vi "EXDIR-YAML_Parse_Exdir.vi"() -> ()   [LabVIEW 2016]
uses:
  <vilib>/NI/Tree/Tree Manager/Tree.lvclass
panel:
  out "substring before match":string
  in  "stop":bool
  in  "OK":bool
  in  "Tree":string(tree)
  out "text":string
  in  "file (use dialog)":path
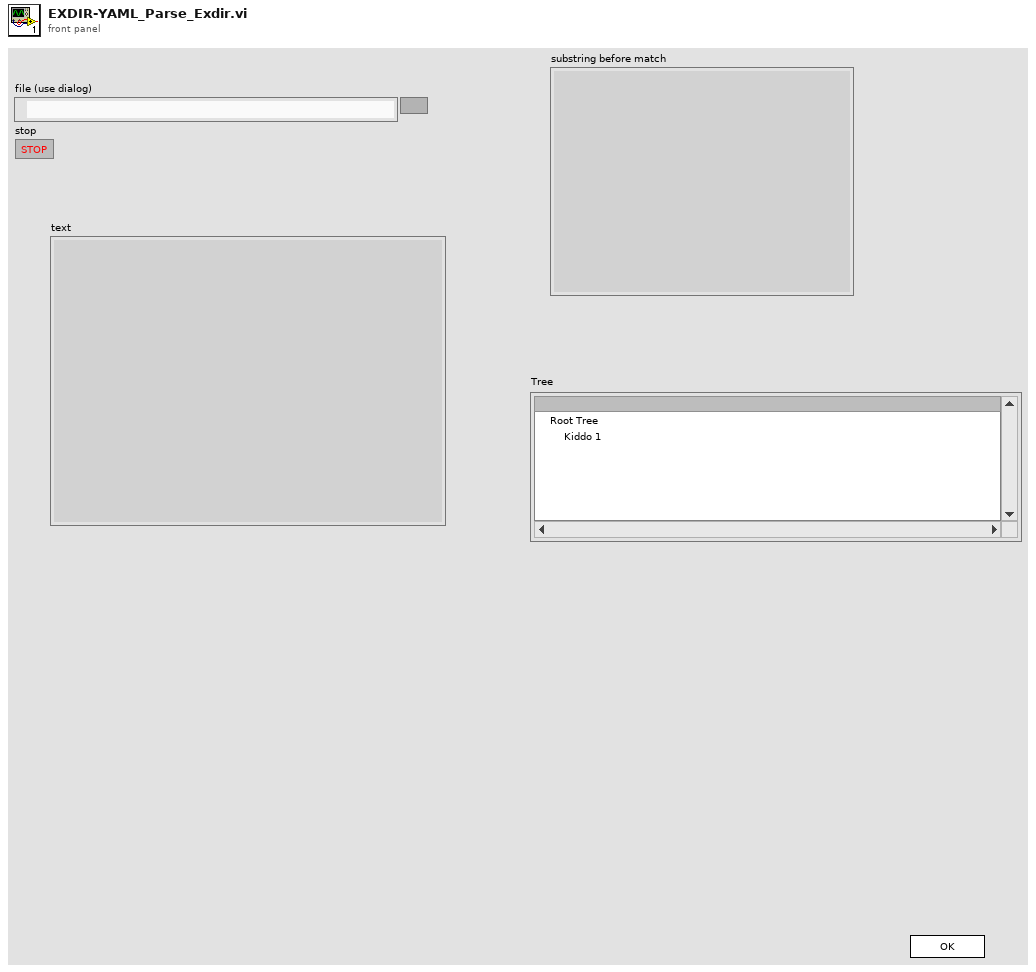
[diagram p1: front panel]
types:
  T1 = enum32{"invalid app kind", "Development System", "Run Time System", "Student Edition", "Embedded LabVIEW", "Evaluation", "Custom"}
  T2 = enum32{"Invalid", "Standard", "Closed", "Hidden", "Minimized", "Maximized"}
  T3 = cluster{"Core":cluster{"Current VI Reference":refnum<vi>, "Close Panel on Exit?":bool}, "Tree Manager":refnum<data-value>, "Unique ID":string, "Value":path, "Full YAML String":string, "queue out":refnum<queue>}
  T4 = cluster{"Current VI Reference":refnum<vi>, "Close Panel on Exit?":bool}
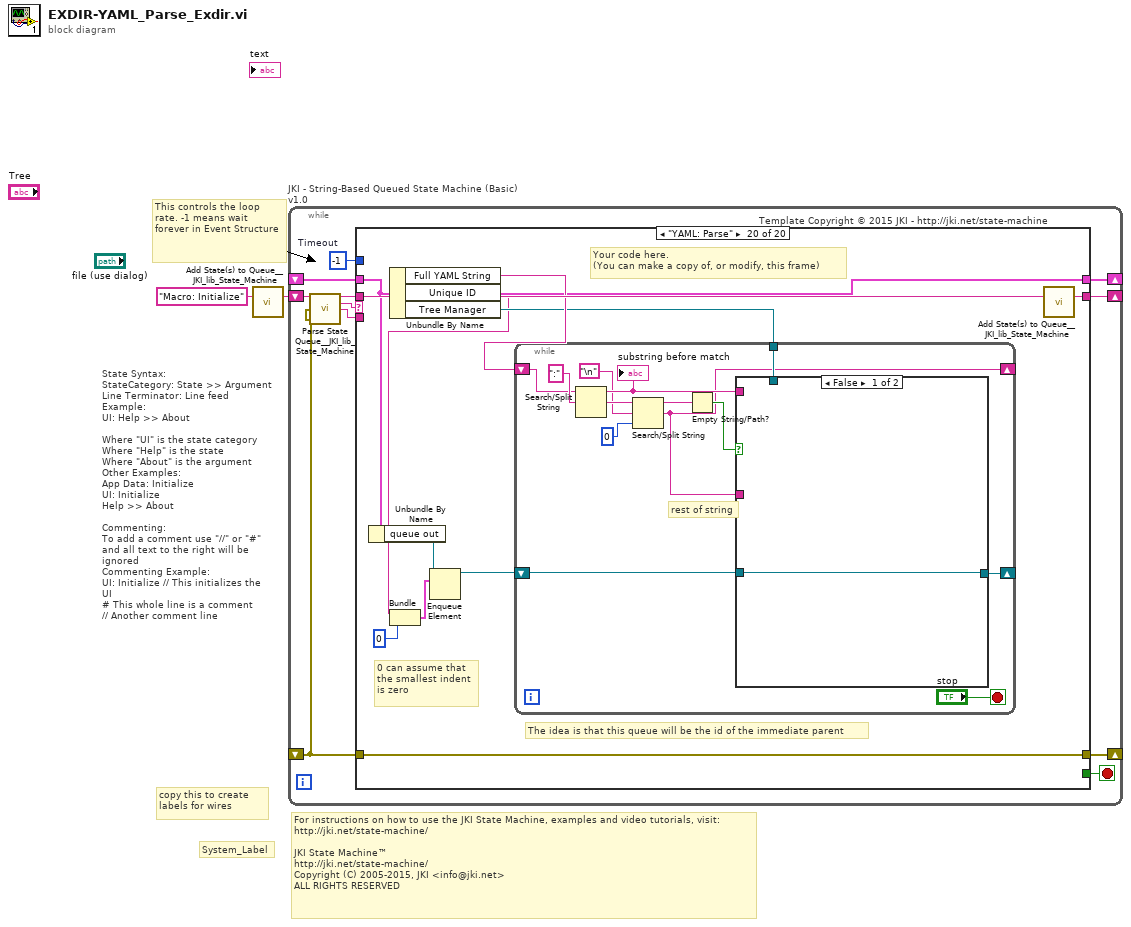
[diagram p0: block diagram]
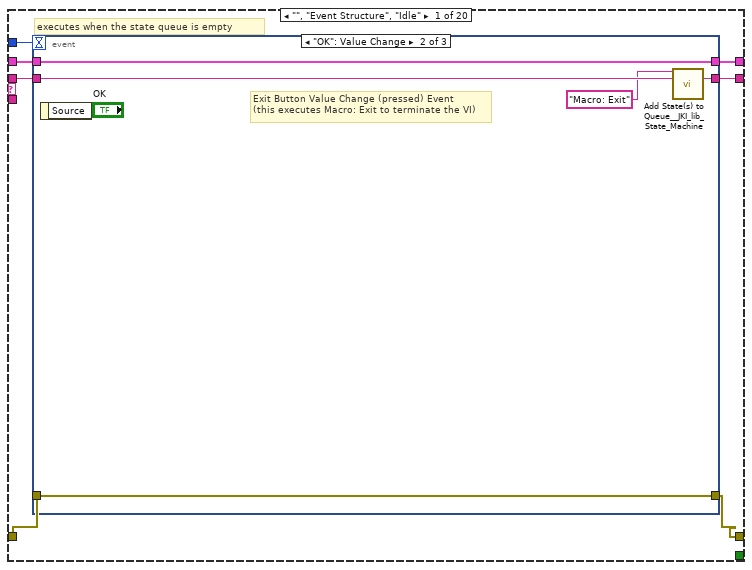
[diagram p2: hidden frame]
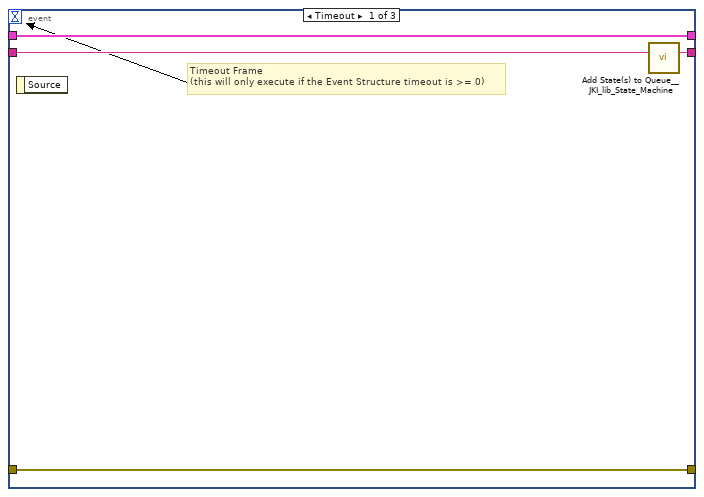
[diagram p3: hidden frame]
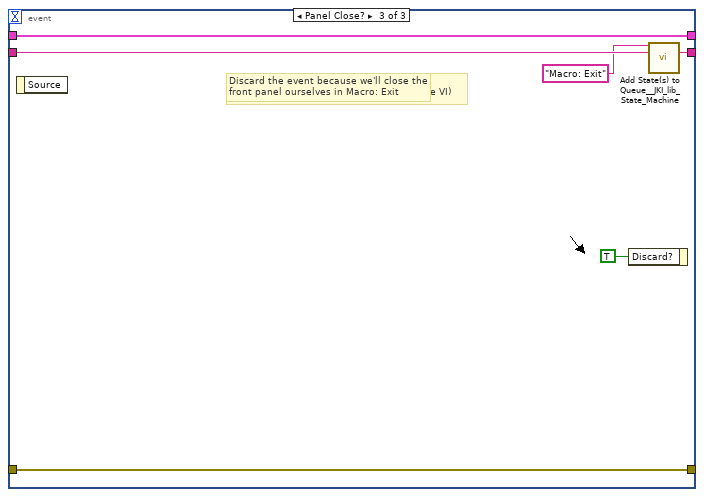
[diagram p4: hidden frame]
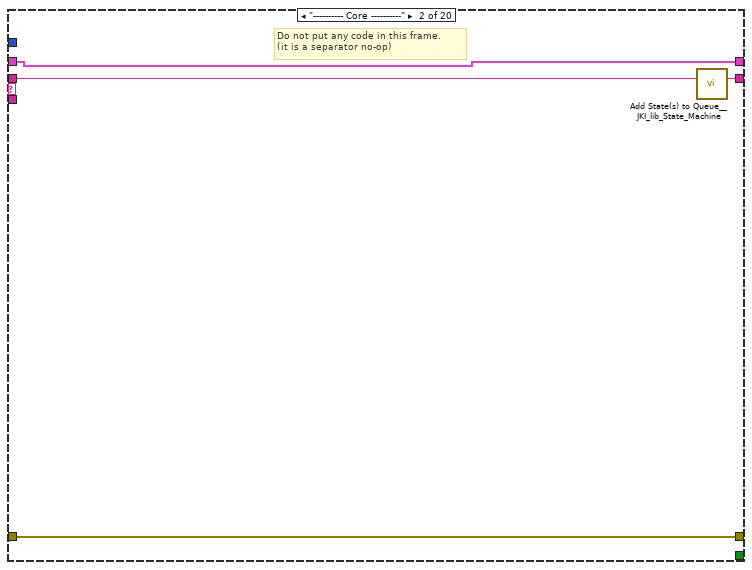
[diagram p5: hidden frame]
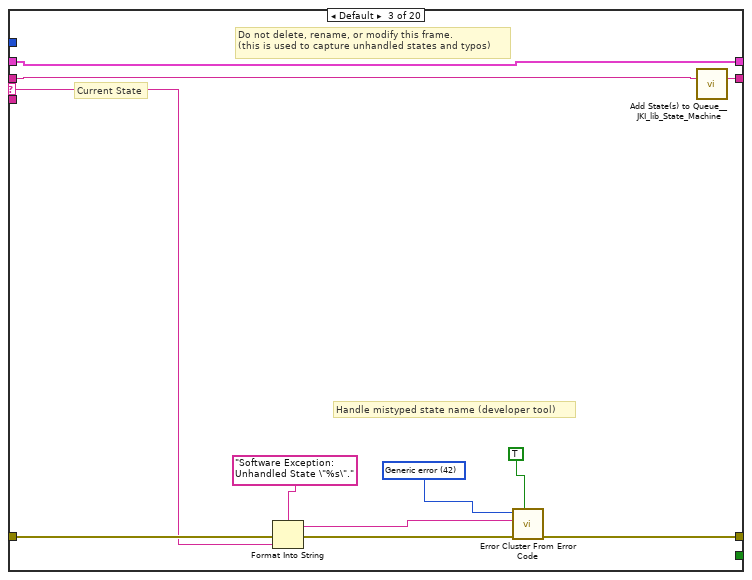
[diagram p6: hidden frame]
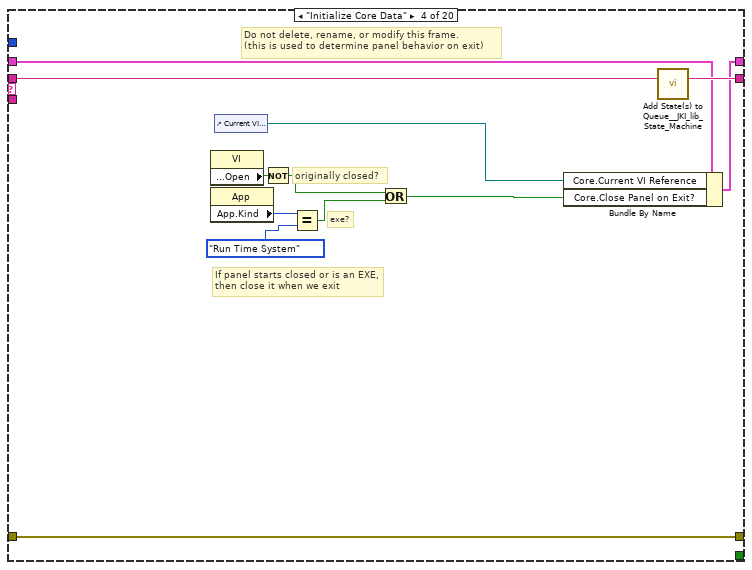
[diagram p7: hidden frame]
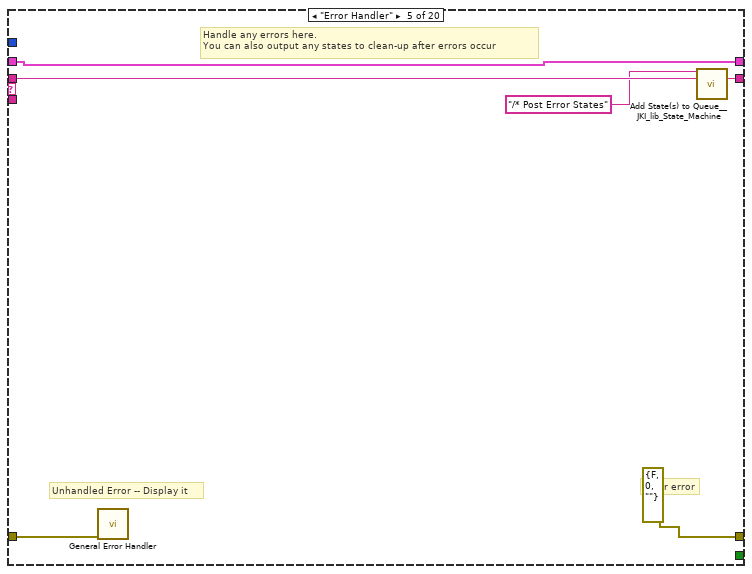
[diagram p8: hidden frame]
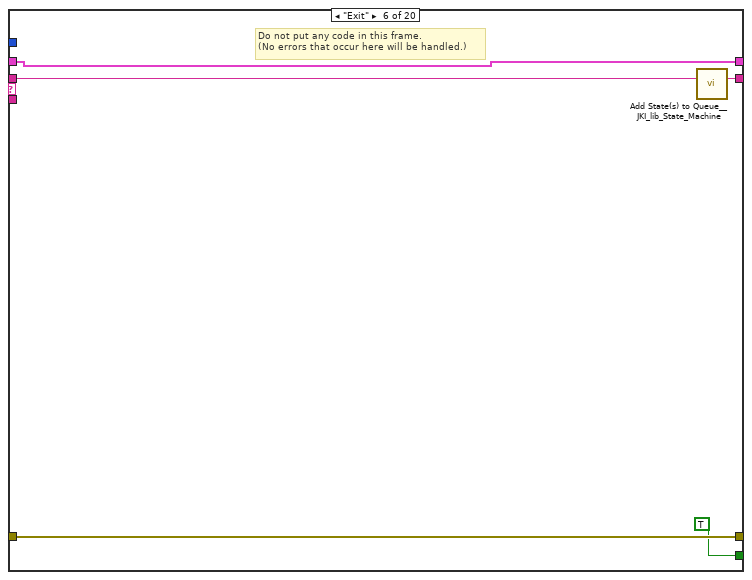
[diagram p9: hidden frame]
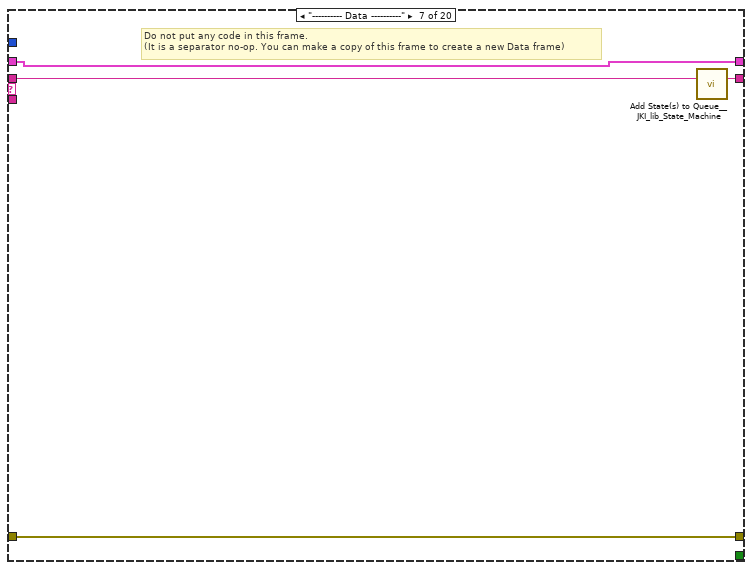
[diagram p10: hidden frame]
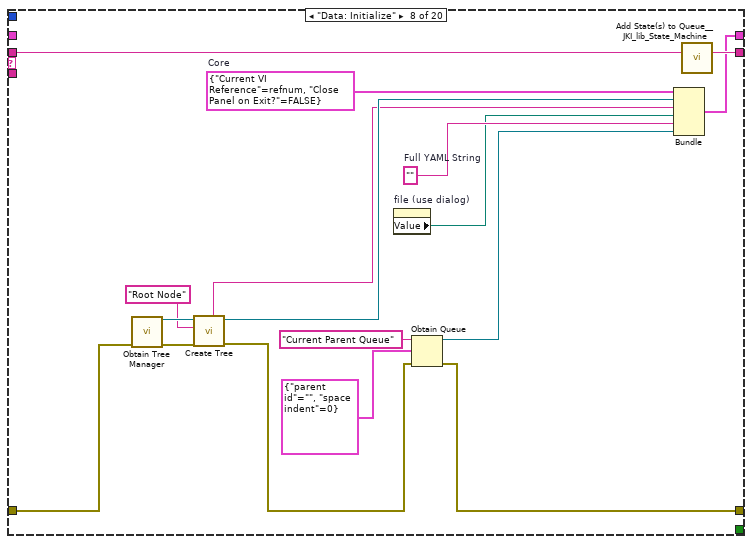
[diagram p11: hidden frame]
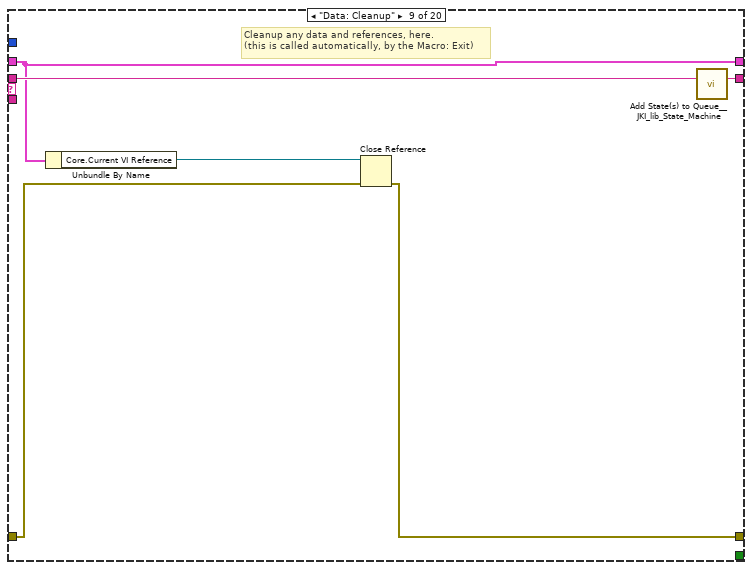
[diagram p12: hidden frame]
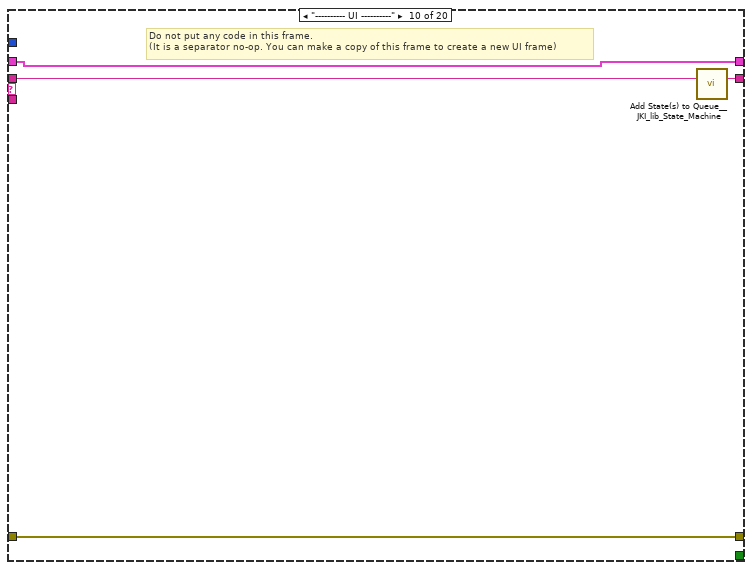
[diagram p13: hidden frame]
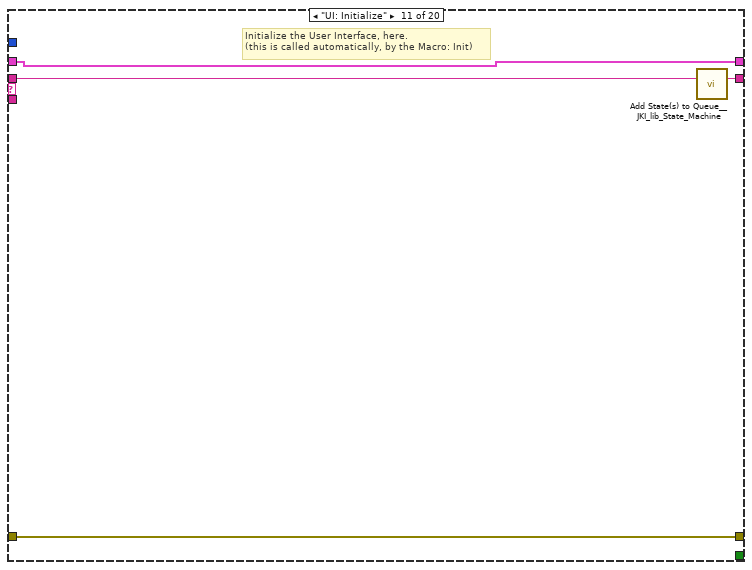
[diagram p14: hidden frame]
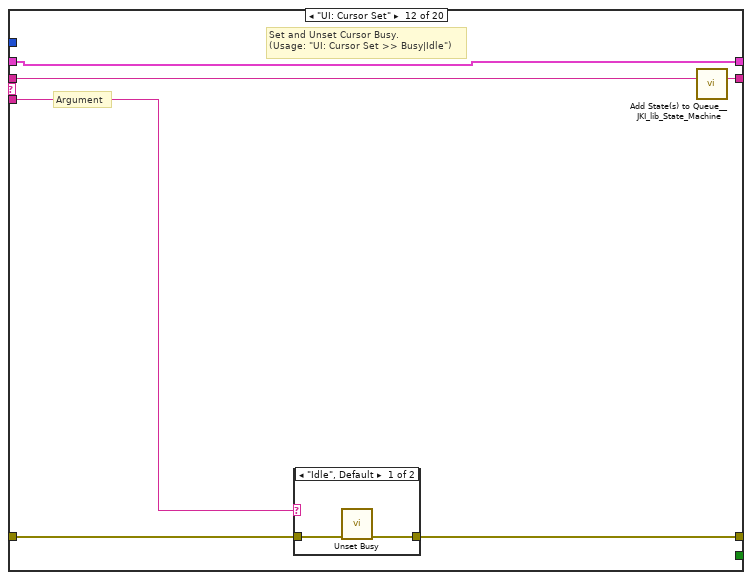
[diagram p15: hidden frame]
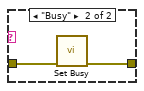
[diagram p16: hidden frame]
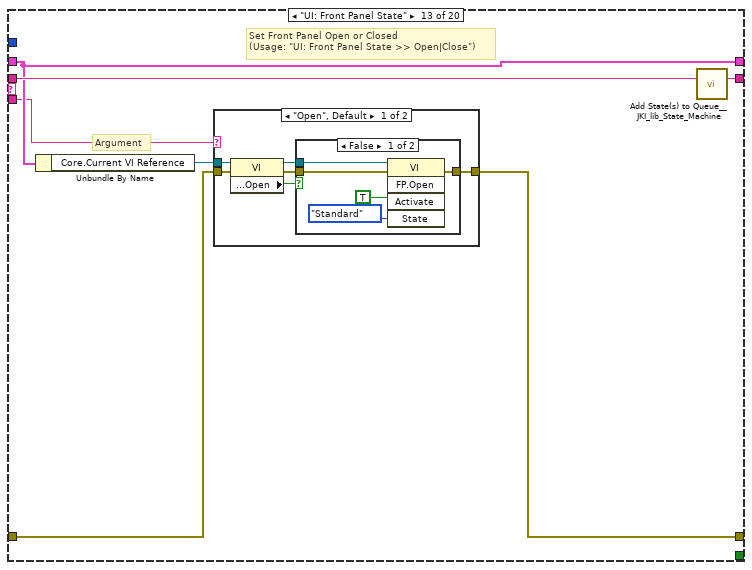
[diagram p17: hidden frame]
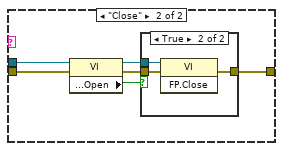
[diagram p19: hidden frame]
diagram:
  # "For instructions on how to use the JKI State Machine, examples and video tutorials, visit:\nhttp://jki.net/state-machine/\n\nJKI State Machine™\nhttp://jki.net/state-machine/\nCopyright (C) 2005-2015, JKI <info@jki.net>\nALL RIGHTS RESERVED"
  # "State Syntax:\nStateCategory: State >> Argument\nLine Terminator: Line feed\nExample:\nUI: Help >> About\n\nWhere \"UI\" is the state category\nWhere \"Help\" is the state\nWhere \"About\" is the argument\nOther Examples:\nApp Data: Initialize\nUI: Initialize\nHelp >> About\n\nCommenting:\nTo add a comment use \"//\" or \"#\" and all text to the right will be ignored\nCommenting Example:\nUI: Initialize // This initializes the UI\n# This whole line is a comment\n// Another comment line"
  # "copy this to create labels for wires"
  # "This controls the loop rate. -1 means wait forever in Event Structure"
  # "System_Label"
  n1 = call <vilib>:"Add State(s) to Queue__JKI_lib_State_Machine.vi"("State(s) in (\"\")"="Macro: Initialize") -> ("States Out"=w2:string)  [unwired: 14 in]
  n2 = while "JKI - String-Based Queued State Machine (Basic) v1.0" {
    shift-right: [w6] -> _
    shift-left: _ -> [w5]
    shift-right: [w9] -> _
    shift-left: _ -> [w3]
    shift-right: [w8] -> _
    shift-left: w2 -> [w10]
    stop <- w7 stop-if-true
    w4 = -1  # Timeout
    # "Template Copyright © 2015 JKI - http://jki.net/state-machine"
    n3 = call <vilib>:"Parse State Queue__JKI_lib_State_Machine.vi"("State Queue"=w10, "Error In (no error)"=w3) -> ("Remaining States"=w12:string, "Current State"=w13:string, "Arguments"=w11:string)  [unwired: 11 in]
    n4 = case shown="\"YAML: Parse\"" w13 {
      selector: w13 -> [_ _ w40 _ _ _ _ _ _ _ _ _ _ _ _ _ _ _ _ _]
      tunnel: w12 -> [w20 w39 w44 w62 w68 w73 w77 w94 w100 w104 w108 w114 w125 w151 w156 w161 w171 w175 w183 w194]
      tunnel: w11 -> [_ _ _ _ _ _ _ _ _ _ _ w109 w119 _ _ _ _ _ _ _]
      tunnel: w5 -> [w18 w36 w42 w53 w65 w71 w74 _ w95 w101 w106 w112 w121 w148 w153 w158 w168 w172 w180 w189]
      tunnel: [w17 w37 w46 w59 errorcluster {"status"=FALSE, "code"=0, "source"=""} ("error out") w70 w75 w81 w96 w102 w105 w110 w122 w149 w154 w159 w169 w173 w176 w192] -> w9
      tunnel: w3 -> [w16 w37 w45 w59 w64 w70 w75 w90 w97 w102 w105 w111 w123 w149 w154 w159 w169 w173 w177 w192]
      tunnel: [w19 w38 w43 w61 w67 w72 w76 w93 w99 w103 w107 w113 w124 w150 w155 w160 w170 w174 w182 w193] -> w8
      tunnel: [_ _ _ _ _ TRUE _ _ _ _ _ _ _ _ _ _ _ _ _ _] -> w7
      tunnel: [w15 w36 w42 w60 w65 w71 w74 w92 w95 w101 w106 w112 w121 w148 w153 w158 w168 w172 w179 w189] -> w6
      tunnel: w4 -> [w14 _ _ _ _ _ _ _ _ _ _ _ _ _ _ _ _ _ _ _]
      frame "", "Event Structure", "Idle" {
        # "executes when the state queue is empty"
        n5 = event shown="[1] \"OK\": Value Change" {
          selector: _ -> [_ _ _]
          dyn-events: _ -> [_ _ _]
          timeout: w14 -> [_ _ _]
          tunnel: w20 -> [w24 w29 w35]
          tunnel: [w23 w28 w34] -> w19
          tunnel: w18 -> [w21 w26 w32]
          tunnel: [w22 w27 w33] -> w17
          tunnel: w16 -> [w22 w27 w33]
          tunnel: [w21 w26 w32] -> w15
          event Timeout {
            # "Timeout Frame\n(this will only execute if the Event Structure timeout is >= 0)"
            n6 = event-data() -> ()  [unwired: 1 in, 1 out]
            n7 = call <vilib>:"Add State(s) to Queue__JKI_lib_State_Machine.vi"("State(s) in (\"\")"=w24) -> ("States Out"=w23:string)  [unwired: 14 in]
          }
          event "OK": Value Change {
            # "Exit Button Value Change (pressed) Event\n(this executes Macro: Exit to terminate the VI)"
            n8 = event-data() -> ()  [unwired: 1 in, 1 out]
            n9 = call <vilib>:"Add State(s) to Queue__JKI_lib_State_Machine.vi"("State(s) in Front (\"\")"="Macro: Exit", "State(s) in (\"\")"=w29) -> ("States Out"=w28:string)  [unwired: 13 in]
          }
          event Panel Close? {
            # "Discard the event because we'll close the front panel ourselves in Macro: Exit"
            # "Close Panel button (pressed) Event\n(this executes Macro: Exit to terminate the VI)"
            n10 = event-data() -> ()  [unwired: 1 in, 1 out]
            n11 = event-data("Discard?"=TRUE) -> ()  [unwired: 1 in, 1 out]
            n12 = call <vilib>:"Add State(s) to Queue__JKI_lib_State_Machine.vi"("State(s) in Front (\"\")"="Macro: Exit", "State(s) in (\"\")"=w35) -> ("States Out"=w34:string)  [unwired: 13 in]
          }
        }
      }
      frame "---------- Core ----------" {
        # "Do not put any code in this frame.\n(it is a separator no-op)"
        n13 = call <vilib>:"Add State(s) to Queue__JKI_lib_State_Machine.vi"("State(s) in (\"\")"=w39) -> ("States Out"=w38:string)  [unwired: 14 in]
      }
      frame Default {
        w49 = 42 items=["No error", "Argument error", "Memory is full", "Out of zone", "End of file", "File already open", "Generic file I/O error", "File not found", "File permission error", "Disk is full", "Duplicate path", "Too many files open", "System feature not enabled", "Resource file not found", "Cannot add resource", "Resource not found", "Image not found", "Image memory error", "Pen does not exist", "Config type invalid", "Config token not found", "Config parse error", "Config memory error", "Bad external code format", "Bad external code offset", "External code not present", "Null window", "Destroy window error", "Null menu", "Print aborted", "Bad print record", "Print driver error", "Windows error during printing", "Memory error during printing", "Print dialog error", "Generic print error", "Invalid device refnum", "Device not found", "Device parameter error", "Device unit error", "Cannot open device", "Device call aborted", "Generic error", "Cancelled by user", "Object ID too low", "Object ID too high", "Object not in heap", "Unknown heap", "Unknown object (invalid DefProc)", "Unknown object (DefProc not in table)", "Message out of range", "Invalid (null) method", "Unknown message", "Manager call not supported", "Bad address", "Network operation in progress", "Network operation timed out", "Connection is busy", "Network attribute not supported", "Network error", "Address in use", "System out of memory", "Connection aborted", "Connection refused", "Not connected", "Already connected", "Connection closed", "Initialization error (interapplication manager)", "Bad occurrence", "Wait on unbound occurrence handler", "Occurrence queue overflow", "Datalog type conflict", "Unused", "Unrecognized type (interapplication manager)", "Memory corrupt", "Failed to make temporary DLL", "Old CIN version", "Drag socket not found", "Failed to load drop-object", "Failed to register OLE object", "Failed to release OLE object", "Format specifier type mismatch", "Unknown format specifier", "Too few format specifiers", "Too many format specifiers", "Scan failed", "Newer CIN version", "Error converting to variant", "Runtime menu error", "Password tampered", "Variant attribute not found", "Incompatible variant data type", "Event data is not available", "Event Store is not present", "Occurrence is not found", "Event Queue is not created", "Event info is not available", "Refnum passed is NULL", "Error retrieving Class GUID", "Error retrieving CoClass GUID", "Error retrieving TypeLib GUID.", "Bad built application magic bytes.", "Specific driver is different from the specific driver associated with the Logical Name.", "There is no session opened to the class driver.", "Max Error", "MAX - Error with config objects", "MAX - Error loading configuration", "MAX - Group not supported"]
        # "Current State"
        # "Do not delete, rename, or modify this frame.\n(this is used to capture unhandled states and typos)"
        # "Handle mistyped state name (developer tool)"
        n14 = Format Into String(format string="Software Exception: Unhandled State \"%s\"." ("message"), error in=w45, w40) -> (resulting string=w48:string, error out=w47:errorcluster)  [unwired: 1 in]
        n15 = call <vilib>:"Error Cluster From Error Code.vi"("show call chain? (False)"=TRUE, "error in (no error)"=w47, "error message (\"\")"=w48, "error code (0)"=w49) -> ("error out"=w46:errorcluster)  [unwired: 5 in]
        n16 = call <vilib>:"Add State(s) to Queue__JKI_lib_State_Machine.vi"("State(s) in (\"\")"=w44) -> ("States Out"=w43:string)  [unwired: 14 in]
      }
      frame "Initialize Core Data" {
        # "Do not delete, rename, or modify this frame.\n(this is used to determine panel behavior on exit)"
        # "originally closed?"
        # "exe?"
        # "If panel starts closed or is an EXE, then close it when we exit"
        n17 = property class="VI"() -> ("Front Panel.Open"=w58:bool)  [unwired: 2 in, 2 out]
        n18 = property class="App"() -> ("App.Kind"=w57:T1)  [unwired: 2 in, 2 out]
        n19 = control-ref of="Current VI Reference"() -> (w51:refnum<vi>)
        n20 = Not(x=w58) -> (.not. x?=w55:bool)
        n21 = Equal?(x=w57, y=T1."Run Time System" ("Application:Kind")) -> (x = y?=w54:bool)
        n22 = Or(x=w55, y=w54) -> (x .or. y?=w52:bool)
        n23 = Bundle By Name(cluster=w53, "Core.Current VI Reference"=w51, "Core.Close Panel on Exit?"=w52) -> (w60:T3)
        n24 = call <vilib>:"Add State(s) to Queue__JKI_lib_State_Machine.vi"("State(s) in (\"\")"=w62) -> ("States Out"=w61:string)  [unwired: 14 in]
      }
      frame "Error Handler" {
        # "Unhandled Error -- Display it"
        # "Handle any errors here.\nYou can also output any states to clean-up after errors occur"
        # "Clear error"
        n25 = call <vilib>:"General Error Handler.vi"("error in (no error)"=w64) -> ()  [unwired: 10 in, 5 out]
        n26 = call <vilib>:"Add State(s) to Queue__JKI_lib_State_Machine.vi"("State(s) in Front (\"\")"="/* Post Error States", "State(s) in (\"\")"=w68) -> ("States Out"=w67:string)  [unwired: 13 in]
      }
      frame "Exit" {
        # "Do not put any code in this frame.\n(No errors that occur here will be handled.)"
        n27 = call <vilib>:"Add State(s) to Queue__JKI_lib_State_Machine.vi"("State(s) in (\"\")"=w73) -> ("States Out"=w72:string)  [unwired: 14 in]
      }
      frame "---------- Data ----------" {
        # "Do not put any code in this frame.\n(It is a separator no-op. You can make a copy of this frame to create a new Data frame)"
        n28 = call <vilib>:"Add State(s) to Queue__JKI_lib_State_Machine.vi"("State(s) in (\"\")"=w77) -> ("States Out"=w76:string)  [unwired: 14 in]
      }
      frame "Data: Initialize" {
        w89 = ""  # Full YAML String
        w91 = T4 {"Current VI Reference"=refnum, "Close Panel on Exit?"=FALSE}  # Core
        n29 = call <vilib>:"Obtain Tree Manager.vi"("Error In"=w90) -> ("Error Out"=w86:errorcluster, "Tree"=w88:refnum<data-value>)  [unwired: 9 in]
        n30 = call <vilib>:"Create Tree.vi"("Error In"=w86, "Name"="Root Node", "Tree Manager"=w88) -> ("Error Out"=w82:errorcluster, "Tree Manager"=w87:refnum<data-value>, "Unique ID"=w84:string)  [unwired: 6 in]
        n31 = property on="file (use dialog)" class="Path"() -> ("Value"=w79:path)  [unwired: 2 in, 2 out]
        n32 = Obtain Queue(name (unnamed)="Current Parent Queue", element data type=cluster{"parent id":string, "space indent":i32} {"parent id"="", "space indent"=0}, error in (no error)=w82) -> (queue out=w80:refnum<queue>, error out=w81:errorcluster)  [unwired: 2 in, 1 out]
        n33 = Bundle("Core"=w91, "Tree Manager"=w87, "Unique ID"=w84, "Value"=w79, "Full YAML String"=w89, "queue out"=w80) -> (w92:T3)  [unwired: 1 in]
        n34 = call <vilib>:"Add State(s) to Queue__JKI_lib_State_Machine.vi"("State(s) in (\"\")"=w94) -> ("States Out"=w93:string)  [unwired: 14 in]
      }
      frame "Data: Cleanup" {
        # "Cleanup any data and references, here.\n(this is called automatically, by the Macro: Exit)"
        n35 = Unbundle By Name(w95) -> ("Core.Current VI Reference"=w98:refnum<vi>)
        n36 = Close Reference(reference=w98, error in (no error)=w97) -> (error out=w96:errorcluster)
        n37 = call <vilib>:"Add State(s) to Queue__JKI_lib_State_Machine.vi"("State(s) in (\"\")"=w100) -> ("States Out"=w99:string)  [unwired: 14 in]
      }
      frame "---------- UI ----------" {
        # "Do not put any code in this frame.\n(It is a separator no-op. You can make a copy of this frame to create a new UI frame)"
        n38 = call <vilib>:"Add State(s) to Queue__JKI_lib_State_Machine.vi"("State(s) in (\"\")"=w104) -> ("States Out"=w103:string)  [unwired: 14 in]
      }
      frame "UI: Initialize" {
        # "Initialize the User Interface, here.\n(this is called automatically, by the Macro: Init)"
        n39 = call <vilib>:"Add State(s) to Queue__JKI_lib_State_Machine.vi"("State(s) in (\"\")"=w108) -> ("States Out"=w107:string)  [unwired: 14 in]
      }
      frame "UI: Cursor Set" {
        # "Argument"
        # "Set and Unset Cursor Busy.\n(Usage: \"UI: Cursor Set >> Busy|Idle\")"
        n40 = case shown="\"Idle\", Default" w109 {
          tunnel: w111 -> [w116 w118]
          tunnel: [w115 w117] -> w110
          frame "Idle", Default {
            n41 = call <vilib>:"Unset Busy.vi"("error in (no error)"=w116) -> ("error out"=w115:errorcluster)  [unwired: 10 in]
          }
          frame "Busy" {
            n42 = call <vilib>:"Set Busy.vi"("error in (no error)"=w118) -> ("error out"=w117:errorcluster)  [unwired: 9 in, 1 out]
          }
        }
        n43 = call <vilib>:"Add State(s) to Queue__JKI_lib_State_Machine.vi"("State(s) in (\"\")"=w114) -> ("States Out"=w113:string)  [unwired: 14 in]
      }
      frame "UI: Front Panel State" {
        # "Argument"
        # "Set Front Panel Open or Closed\n(Usage: \"UI: Front Panel State >> Open|Close\")"
        n44 = Unbundle By Name(w121) -> ("Core.Current VI Reference"=w120:refnum<vi>)
        n45 = case shown="\"Open\", Default" w119 {
          tunnel: w123 -> [w129 w142]
          tunnel: [w131 w143] -> w122
          tunnel: w120 -> [w130 w140]
          frame "Open", Default {
            n46 = property class="VI"(reference=w130, error in=w129) -> (reference out=w127:refnum<vi>, error out=w128:errorcluster, "Front Panel.Open"=w126:bool)
            n47 = case shown="False" w126 {
              tunnel: [w134 w137] -> w131
              tunnel: w128 -> [w133 w137]
              tunnel: w127 -> [w132 _]
              frame False {
                n48 = invoke class="VI" method="FP.Open"(reference=w132, error in=w133, "Activate"=TRUE, "State"=T2."Standard") -> (error out=w134:errorcluster)  [unwired: 1 in, 4 out]
              }
              frame True {
              }
            }
          }
          frame "Close" {
            n49 = property class="VI"(reference=w140, error in=w142) -> (reference out=w139:refnum<vi>, error out=w141:errorcluster, "Front Panel.Open"=w138:bool)
            n50 = case shown="True" w138 {
              tunnel: [w144 w147] -> w143
              tunnel: w141 -> [w144 w146]
              tunnel: w139 -> [_ w145]
              frame False {
              }
              frame True {
                n51 = invoke class="VI" method="FP.Close"(reference=w145, error in=w146) -> (error out=w147:errorcluster)  [unwired: 1 in, 2 out]
              }
            }
          }
        }
        n52 = call <vilib>:"Add State(s) to Queue__JKI_lib_State_Machine.vi"("State(s) in (\"\")"=w125) -> ("States Out"=w124:string)  [unwired: 14 in]
      }
      frame "---------- Macro ----------" {
        # "Do not put any code in this frame.\n(It is a separator no-op. You can make a copy of this frame to create a new Macro frame)"
        n53 = call <vilib>:"Add State(s) to Queue__JKI_lib_State_Machine.vi"("State(s) in (\"\")"=w151) -> ("States Out"=w150:string)  [unwired: 14 in]
      }
      frame "Macro: Initialize" {
        w152 = "Data: Initialize\nInitialize Core Data\nUI: Initialize\nUI: Front Panel State >> Open\nYAML: Read File\nYAML: Parse"  # Data: Initialize Initialize Core Data UI: Initialize UI: Front Panel State >> Open YAML: Read File YAML: Parse
        # "Initialization Macro\n(This is called once, when the VI starts)"
        n54 = call <vilib>:"Add State(s) to Queue__JKI_lib_State_Machine.vi"("State(s) in Front (\"\")"=w152, "State(s) in (\"\")"=w156) -> ("States Out"=w155:string)  [unwired: 13 in]
      }
      frame "Macro: Parse YAML String" {
        # "Initialization Macro\n(This is called once, when the VI starts)"
        n55 = call <vilib>:"Add State(s) to Queue__JKI_lib_State_Machine.vi"("State(s) in Front (\"\")"="YAML: ", "State(s) in (\"\")"=w161) -> ("States Out"=w160:string)  [unwired: 13 in]
      }
      frame "Macro: Exit" {
        # "Exit Macro\n(This is called once, when the VI exits)"
        n56 = Unbundle By Name(w168) -> ("Core.Close Panel on Exit?"=w167:bool)
        n57 = Select(t="UI: Front Panel State >> Close", s=w167, f="") -> (s? t:f=w164:string)
        n58 = call <vilib>:"Add State(s) to Queue__JKI_lib_State_Machine.vi"("State(s) in (\"\")"=w164, "State(s) at Back (\"\")"="Data: Cleanup\nExit") -> ("States Out"=w162:string)  [unwired: 13 in]
        n59 = call <vilib>:"Add State(s) to Queue__JKI_lib_State_Machine.vi"("State(s) in Front (\"\")"=w162, "State(s) in (\"\")"=w171) -> ("States Out"=w170:string)  [unwired: 13 in]
      }
      frame "---------- YAML ----------" {
        # "Template Separator\n(You can make a copy of, or modify, this frame)"
        n60 = call <vilib>:"Add State(s) to Queue__JKI_lib_State_Machine.vi"("State(s) in (\"\")"=w175) -> ("States Out"=w174:string)  [unwired: 14 in]
      }
      frame "YAML: Read File" {
        n61 = Unbundle By Name(w180) -> ("Value"=w181:path)
        n62 = Read from Text File(file (use dialog)=w181, error in=w177) -> (text=w178:string, error out=w176:errorcluster)  [unwired: 2 in, 2 out]
        n63 = Bundle By Name(cluster=w180, "Full YAML String"=w178) -> (w179:T3)
        n64 = call <vilib>:"Add State(s) to Queue__JKI_lib_State_Machine.vi"("State(s) in (\"\")"=w183) -> ("States Out"=w182:string)  [unwired: 14 in]
      }
      frame "YAML: Parse" {
        # "0 can assume that \nthe smallest indent\nis zero"
        # "The idea is that this queue will be the id of the immediate parent"
        # "Your code here.\n(You can make a copy of, or modify, this frame)"
        n65 = Unbundle By Name(w189) -> ("queue out"=w188:refnum<queue>)
        n66 = Unbundle By Name(w189) -> ("Full YAML String"=w191:string, "Unique ID"=w186:string, "Tree Manager"=w190:refnum<data-value>)
        n67 = Bundle("Unique ID"=w186, 0) -> (w184:cluster{"Unique ID":string, i32})  [unwired: 1 in]
        n68 = Enqueue Element(queue=w188, element=w184) -> (queue out=w187:refnum<queue>)  [unwired: 2 in, 2 out]
        n69 = while {
          shift-right: [w195] -> _
          shift-left: w191 -> [w206]
          tunnel: w190 -> [w201]
          shift-right: [w198] -> _
          shift-left: w187 -> [w199]
          stop <- "stop" stop-if-true
          # "rest of string"
          n70 = Search/Split String(string=w206, search string/char (-)=":") -> (substring before match=w203:string, match + rest of string=w204:string)  [unwired: 1 in, 1 out]
          "substring before match" <- w203
          n71 = Search/Split String(string=w204, search string/char (-)="\n", offset (0)=0) -> (substring before match=w197:string, match + rest of string=w195:string)  [unwired: 1 out]
          n72 = Empty String/Path?(string/path=w197) -> (empty?=w202:bool)
          n73 = case shown="False" w202 {
            tunnel: w203 -> [_ w219]
            tunnel: w201 -> [_ w220]
            tunnel: w199 -> [w208 w218]
            tunnel: [w208 w216] -> w198
            tunnel: w195 -> [_ w210]
            frame False {
            }
            frame True {
              # "need to know the # of indents"
              # "Empty here means the pre-colon string\nwas a container, so make it a parent"
              n74 = Preview Queue Element(queue=w218) -> (queue out=w217:refnum<queue>, element=w215:cluster{"parent id":string, "space indent":i32})  [unwired: 2 in, 2 out]
              n75 = Unbundle By Name(w215) -> ("parent id"=w214:string)
              n76 = call <vilib>:"Create Tree.vi"("Parent ID (empty)"=w214, "Name"=w219, "Tree Manager"=w220) -> ("Unique ID"=w213:string)  [unwired: 6 in, 2 out]
              n77 = call "EXDIR-YAML_CountSpaces.vi"(10:1 ("offset"), "String"=w210) -> ("Numeric"=w211:i32)  [unwired: 9 in]
              n78 = Bundle("Unique ID"=w213, "Numeric"=w211) -> (w212:cluster{"Unique ID":string, "Numeric":i32})  [unwired: 1 in]
              n79 = Enqueue Element(queue=w217, element=w212) -> (queue out=w216:refnum<queue>)  [unwired: 2 in, 2 out]
            }
          }
        }
        n80 = call <vilib>:"Add State(s) to Queue__JKI_lib_State_Machine.vi"("State(s) in (\"\")"=w194) -> ("States Out"=w193:string)  [unwired: 14 in]
      }
    }
  }
